vi "post-4616-1160681060.vi"(0 "Pie Chart Data (arb unit)":dbl[](array[numeric]), 5 "Label Text (No Labels)":string[](array[string]), 7 "Division Colors":u32[](array[colorbox]), 9 "Pie Chart Size (200 pixels)":dbl=200.0, 11 "Show Labels (On)":bool=TRUE, 12 "Label Format (text)":T1(ring)=enum."Text labels", 13 "Decimals (2)":i16=2, 14 "Position % (61)":dbl=61.0 format="%.2f") -> (8 "Pie Chart":picture)   [LabVIEW 2014]
doc: "Based on the NI example Pie chart.vi in piechart.llb. Major changes: oriented labels; changed default colors; automatically recycles thru colors after the first (by default) 8; defaults to using text labels. NI's documentation is below.\n\nThis example shows how to create a pie chart using the picture control in LabVIEW.\nPie Chart Data % is an array of positive decimals where you can specify the percentage of the pie taken by a specific variable (color). The sum of the numbers in this array should be 100%.\nDivision's Color is an array of colors where you can specify the color of each division of the chart. \nThe size of the pie can be modified by the user using the Pie Chart Size numeric control. \nAdditionally, the user can add labels to each division; configure the format and precision of the numbers; and the position of the label in the division using the controls in the Labels Configuration section."
panel:
  # "For details see File >> VI Properties >> Documentation."
  # "Labels Configuration"
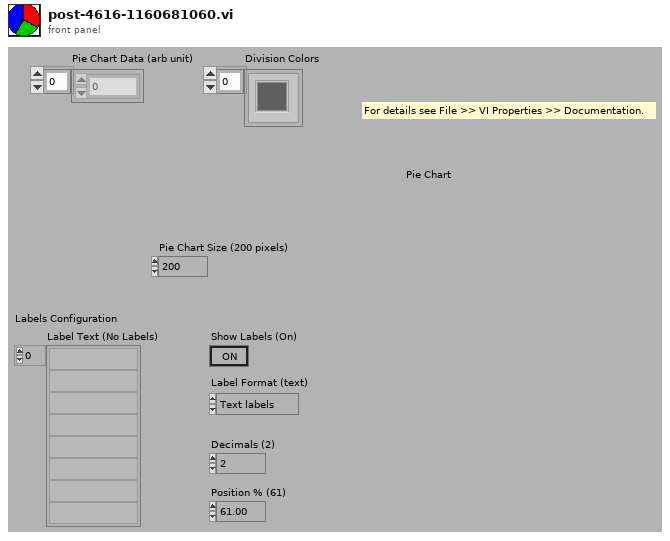
[diagram p1: front panel]
types:
  T1 = enum16{"Engineering", "Fractional", "Exponential", "Text labels"}
  T2 = cluster{"horizontal":enum16{"left", "center", "right"}, "vertical":enum16{"top", "center", "bottom"}}
  T3 = cluster{"left":i16, "top":i16, "right":i16, "bottom":i16}
  T4 = cluster{"Pie Chart Size (200 pixels)":dbl, "Pie Chart Size (200 pixels)":dbl}
  T5 = enum16{"None", "Stacked", "Clockwise", "Counterclockwise"}
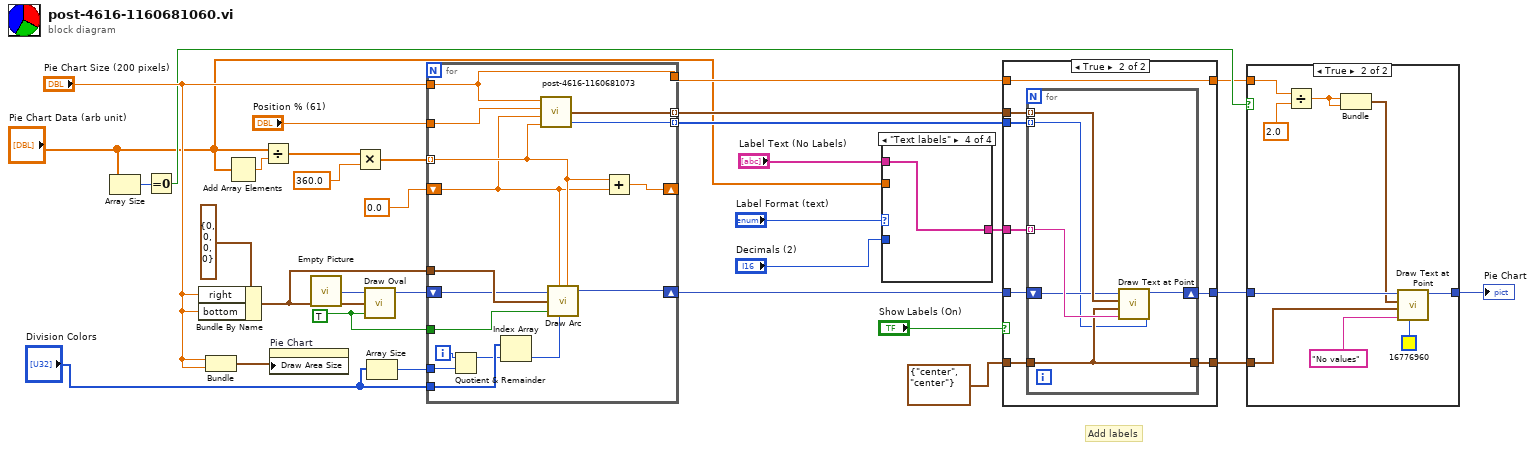
[diagram p0: block diagram]
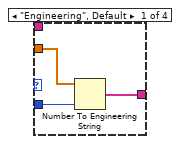
[diagram p3: hidden frame]
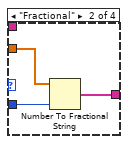
[diagram p4: hidden frame]
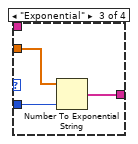
[diagram p5: hidden frame]
diagram:
  w30 = TRUE ("fill?(F)")
  # "Add labels"
  n1 = Array Size(array="Pie Chart Data (arb unit)") -> (size(s)=w12:i32)
  n2 = Equal To 0?(x=w12) -> (x = 0?=w11:bool)
  n3 = Bundle By Name(cluster=T3 {"left"=0, "top"=0, "right"=0, "bottom"=0} ("rect"), "right"="Pie Chart Size (200 pixels)", "bottom"="Pie Chart Size (200 pixels)") -> (w27:T3)
  n4 = Bundle("Pie Chart Size (200 pixels)"="Pie Chart Size (200 pixels)", "Pie Chart Size (200 pixels)"="Pie Chart Size (200 pixels)") -> (w25:T4)  [unwired: 1 in]
  n5 = Add Array Elements(numeric array="Pie Chart Data (arb unit)") -> (sum=w29:dbl)
  n6 = Divide(x="Pie Chart Data (arb unit)", y=w29) -> (x/y=w22:dbl[])
  n7 = property on="Pie Chart" class="Pict"("Draw Area Size"=w25) -> ()  [unwired: 2 in, 2 out]
  n8 = call "Empty Picture"() -> ("empty picture"=w32:picture)
  n9 = Multiply(x=w22, y=360.0) -> (x*y=w23:dbl[])
  n10 = call <vilib>:"Draw Oval.vi"("picture"=w32, "rect"=w27, "fill?(F)"=w30) -> ("new picture"=w26:picture)  [unwired: 6 in]
  n11 = Array Size(array="Division Colors") -> (size(s)=w3:i32)
  n12 = for {
    tunnel: w30 -> [w48]
    tunnel: w23 -> [w43] mode=indexing
    shift-right: [w47] -> _
    shift-left: 0.0 -> [w42]
    tunnel: w27 -> [w46]
    tunnel: "Division Colors" -> [w35]
    shift-right: [w41] -> w16
    shift-left: w26 -> [w45]
    tunnel: "Pie Chart Size (200 pixels)" -> [w39]
    tunnel: [w44] -> w15 mode=indexing
    tunnel: "Position % (61)" -> [w40]
    tunnel: [w39] -> w8
    tunnel: [w38] -> w4 mode=indexing
    tunnel: w3 -> [w36]
    i -> [w37]
    n13 = Quotient & Remainder(x=w37, y=w36) -> (x-y*floor(x/y)=w33:i32)  [unwired: 1 out]
    n14 = Index Array(array=w35, index=w33) -> (element=w34:u32)
    n15 = call "post-4616-1160681073.vi"("New angle"=w43, "Previous angle"=w42, "Position % (50)"=w40, "Width"=w39) -> ("text orientation"=w38:T5, "Origin"=w44:cluster{dbl, dbl})  [unwired: 1 in]
    n16 = call <vilib>:"Draw Arc.vi"("picture"=w45, "start angle[degrees]"=w42, "rect"=w46, "fill?(F)"=w48, "color(black)"=w34, "arc size[degrees]"=w43) -> ("new picture"=w41:picture)  [unwired: 3 in]
    n17 = Add(x=w43, y=w42) -> (x+y=w47:dbl)
  }
  n18 = case shown="\"Text labels\"" "Label Format (text)" {
    tunnel: [w51 w54 w57 w58] -> w28
    tunnel: "Decimals (2)" -> [w50 w53 w56 _]
    tunnel: "Pie Chart Data (arb unit)" -> [w49 w52 w55 _]
    tunnel: "Label Text (No Labels)" -> [_ _ _ w58]
    frame "Engineering", Default {
      n19 = Number To Engineering String(2:w50, 4:w49) -> (0:w51:string[])  [unwired: 2 in]
    }
    frame "Fractional" {
      n20 = Number To Fractional String(number=w52, precision (6)=w53) -> (F-format string=w54:string[])  [unwired: 2 in]
    }
    frame "Exponential" {
      n21 = Number To Exponential String(number=w55, precision (6)=w56) -> (E-format string=w57:string[])  [unwired: 2 in]
    }
    frame "Text labels" {
    }
  }
  n22 = case shown="True" "Show Labels (On)" {
    tunnel: [w61 w65] -> w10
    tunnel: T2 {"horizontal"=enum."center", "vertical"=enum."center"} ("alignment(left, top)") -> [w59 w69]
    tunnel: w16 -> [w61 w66]
    tunnel: w28 -> [_ w68]
    tunnel: w15 -> [_ w67]
    tunnel: w8 -> [w60 w64]
    tunnel: [w60 w64] -> w7
    tunnel: [w59 w63] -> w6
    tunnel: w4 -> [_ w62]
    frame False {
    }
    frame True {
      n23 = for {
        tunnel: w69 -> [w71]
        tunnel: w68 -> [w74] mode=indexing
        tunnel: w67 -> [w75] mode=indexing
        shift-right: [w72] -> w65
        shift-left: w66 -> [w73]
        tunnel: [w71] -> w63
        tunnel: w62 -> [w70] mode=indexing
        n24 = call <vilib>:"Draw Text at Point.vi"("text orientation"=w70, "text"=w74, "alignment(left, top)"=w71, "origin"=w75, "picture"=w73) -> ("new picture"=w72:picture)  [unwired: 5 in, 1 out]
      }
    }
  }
  n25 = case shown="True" w11 {
    tunnel: w10 -> [w76 w85]
    tunnel: [w76 w84] -> w9
    tunnel: w7 -> [_ w81]
    tunnel: w6 -> [_ w78]
    frame False {
    }
    frame True {
      n26 = Divide(x=w81, y=2.0) -> (x/y=w77:dbl)
      n27 = Bundle(w77, w77) -> (w79:cluster{dbl, dbl})  [unwired: 1 in]
      n28 = call <vilib>:"Draw Text at Point.vi"("text color(black)"=u32 16776960, "text"="No values", "alignment(left, top)"=w78, "origin"=w79, "picture"=w85) -> ("new picture"=w84:picture)  [unwired: 5 in, 1 out]
    }
  }
  "Pie Chart" <- w9
